vi "Query Status Register.vi"(8 "error in":errorcluster, 11 "69X_79X in":refnum<class "6972A.lvclass">) -> (0 "error out":errorcluster, 3 "69X_79X out":refnum<class "6972A.lvclass">)   [LabVIEW 2019, in "6972A.lvlib" / "6972A.lvclass"]
doc: "Child classes must override this VI:\n\nThis VI is the device specific query of the supply's status registers. \nThe return values are: \n\nThe implementation must read status registers and push the status register values to private data for:\nOCP Flag, OVP Flag, Interlock Flag, Output Flag into the private data arrays of the power supply class."
uses:
  Library/6972A.lvclass
  C:/Users/Public/Documents/Development/builds/Instruments/PowerSupply.lvlibp/Library/PowerSupply.lvclass
  builds/Instruments/PowerSupply.lvlibp/Custom Controls/Status_Flags.ctl
  Library/6972A.lvclass/6972A.ctl
  builds/Instruments/PowerSupply.lvlibp/Accessors/Write Status Flags.vi
  <instrlib>/Agilent N6900 N7900 Series/Agilent N6900 N7900 Series.lvlib
  builds/Instruments/PowerSupply.lvlibp/Library/PowerSupply.lvclass
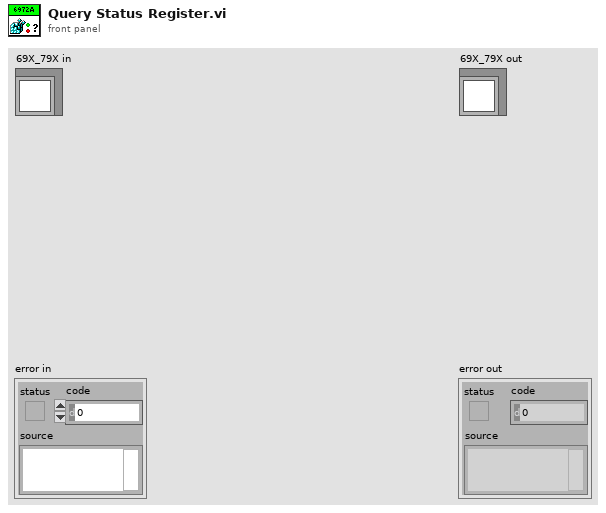
[diagram p1: front panel]
types:
  T1 = typedef "PowerSupply.lvlibp/PowerSupply.lvclass/Status_Flags.ctl" = cluster{"Interlock":bool, "OVP":bool, "OCP":bool, "Output":bool}
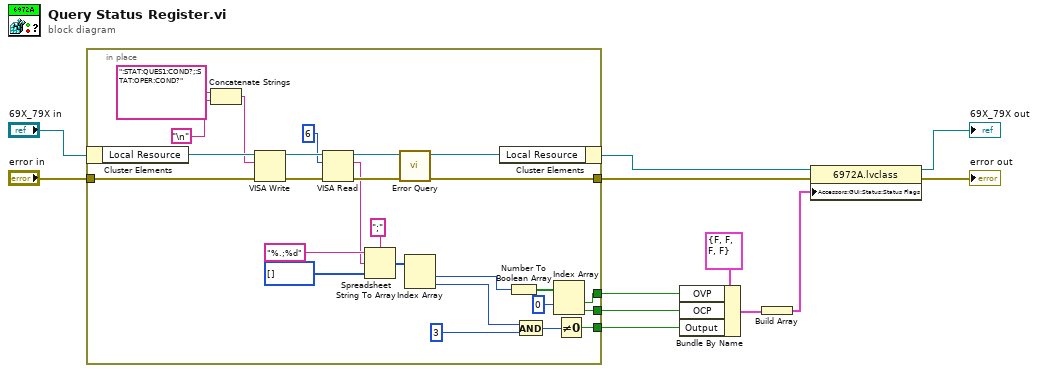
[diagram p0: block diagram]
diagram:
  n1 = in-place {
    in-place-border: "error in" -> [w30]
    in-place-border: [w29] -> w6
    in-place-border: [w19] -> w10
    in-place-border: [w16] -> w8
    in-place-border: [w15] -> w9
    n2 = in-place-cluster #1("69X_79X in") -> ("Local Resource"=w33:refnum<visa-resource-name>)
    n3 = Concatenate Strings(":STAT:QUES1:COND?;:STAT:OPER:COND?", "\n") -> (w14:string)
    n4 = VISA Write(VISA resource name=w33, write buffer=w14, error in (no error)=w30) -> (VISA resource name out=w36:refnum<visa-resource-name>, error out=w35:errorcluster)  [unwired: 1 out]
    n5 = VISA Read(VISA resource name=w36, byte count=u32 6, error in (no error)=w35) -> (VISA resource name out=w37:refnum<visa-resource-name>, read buffer=w25:string, error out=w38:errorcluster)  [unwired: 1 out]
    n6 = Spreadsheet String To Array(delimiter (Tab)=";", format string="%.;%d", spreadsheet string=w25, array type (2D Dbl)=u32[] []) -> (array=w24:u32[])
    n7 = call <instrlib>:"Error Query.vi"("error in (no error)"=w38, "VISA resource name"=w37) -> ("error out"=w29:errorcluster, "VISA resource name out"=w32:refnum<visa-resource-name>)  [unwired: 6 in, 2 out]
    n8 = Index Array(array=w24) -> (element #1=w23:u32, element #2=w22:u32)  [unwired: 2 in]
    n9 = in-place-cluster #1("Local Resource"=w32) -> (w5:refnum<class "6972A.lvclass">)
    n10 = Number To Boolean Array(number=w23) -> (Boolean array=w18:bool[])
    n11 = And(x=w22, y=u32 3 ("x")) -> (x .and. y?=w20:u32)
    n12 = Index Array(array=w18, index #1=0 ("index")) -> (element #1=w16:bool, element #2=w15:bool)  [unwired: 1 in]
    n13 = Not Equal To 0?(x=w20) -> (x != 0?=w19:bool)
  }
  n14 = Bundle By Name(cluster=T1 {"Interlock"=FALSE, "OVP"=FALSE, "OCP"=FALSE, "Output"=FALSE} ("Status"), "OVP"=w8, "OCP"=w9, "Output"=w10) -> (w11:T1)
  n15 = Build Array(w11) -> (w12:T1[])
  n16 = property class="6972A.lvclass"(reference=w5, error in=w6, "Accessors:GUI:Status:Status Flags"=w12) -> (reference out=→"69X_79X out":refnum<class "6972A.lvclass">, error out=→"error out":errorcluster)
